vi "convert_stringArray_to_doubleArray.vi"(2 "Max Elements Count (All)":i32=-1, 3 "default (0)":dbl, 4 "string array in":string[](array[string])) -> (1 "double array out":dbl[](array[numeric]) format="%#.12g")   [LabVIEW 2014, in "rszvl_rsidr_core.lvlib"]
uses:
  rszvl_rsidr_core.lvlib
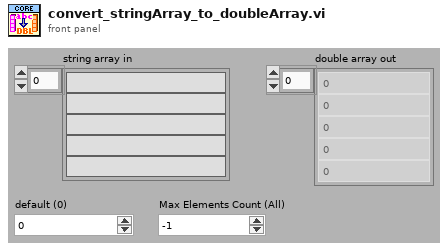
[diagram p1: front panel]
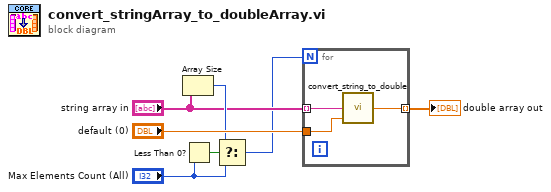
[diagram p0: block diagram]
diagram:
  n1 = Array Size(array="string array in") -> (size(s)=w3:i32)
  n2 = Less Than 0?(x="Max Elements Count (All)") -> (x < 0?=w5:bool)
  n3 = Select(t=w3, s=w5, f="Max Elements Count (All)") -> (s? t:f=w1:i32)
  n4 = for {
    N: w1 -> [_]
    tunnel: "string array in" -> [w10] mode=indexing
    tunnel: [w9] -> w7 mode=indexing
    tunnel: "default (0)" -> [w8]
    n5 = call "convert_string_to_double.vi"("default (0)"=w8, "String in"=w10) -> ("double value out"=w9:dbl)  [unwired: 3 in]
  }
  "double array out" <- w7
